vi "检查前面板控件（使用事件）.vi"() -> ()   [LabVIEW 2010]
uses:
  Instance           2 34Saved   检查前面板控件（使用事件） .vi
  Instance           1 34Saved   检查前面板控件（使用事件） .vi
panel:
  out "波形图":dynamicdata(graph)
  in  "偏移量":dbl(slide)=1.3131313131313131 scale=0.0..5.0
  in  "频率":dbl(slide)=25.757575757575758 scale=0.0..50.0
  in  "幅值":dbl(slide)=5.555555555555555 scale=0.0..10.0
  in  "stop":bool
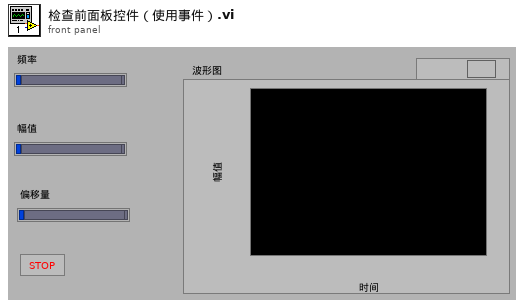
[diagram p1: front panel]
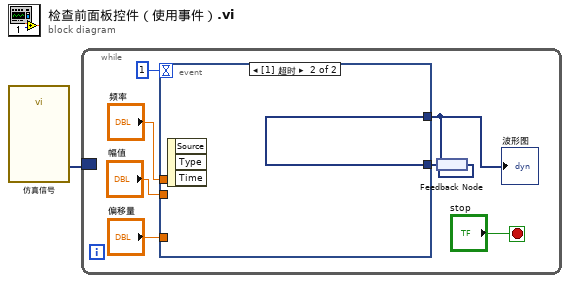
[diagram p0: block diagram]
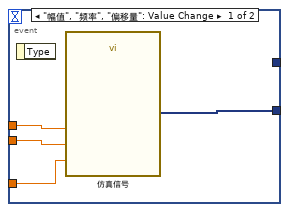
[diagram p2: hidden frame]
diagram:
  n1 = call "仿真信号"() -> ("正弦"=w1:dynamicdata)  [unwired: 14 in, 1 out]
  n2 = while {
    border: w1 -> [_]
    stop <- "stop" stop-if-true
    n3 = feedback #1() -> (w2:dynamicdata)
    "波形图" <- w2
    n4 = event shown="[1] 超时" {
      selector: _ -> [_ _]
      dyn-events: _ -> [_ _]
      timeout: 1 -> [_ _]
      tunnel: [w12 w13] -> w5
      tunnel: "频率" -> [w10 _]
      tunnel: "幅值" -> [w9 _]
      tunnel: "偏移量" -> [w11 _]
      tunnel: w2 -> [_ w13]
      event "幅值", "频率", "偏移量": Value Change {
        n5 = event-data() -> ()  [unwired: 1 in, 1 out]
        n6 = call "仿真信号"("Offset"=w11, "Frequency"=w10, "Amplitude"=w9) -> ("正弦"=w12:dynamicdata)  [unwired: 11 in, 1 out]
      }
      event Timeout {
        n7 = event-data() -> ()  [unwired: 1 in, 3 out]
      }
    }
    n8 = feedback-in #1(w5) -> ()
  }
